vi "Limit range based on sensors.vi"(4 "Position":dbl, 6 "Position Max":dbl, 7 "min speed":dbl=-0.1 format="%#_13g", 8 "BottomDist":dbl=inf, 9 "Bottom SW":bool, 10 "Top SW":bool, 11 "output range in":cluster{"output high":dbl, "output low":dbl}) -> (3 "output range out":cluster{"output high":dbl, "output low":dbl})   [LabVIEW 2019]
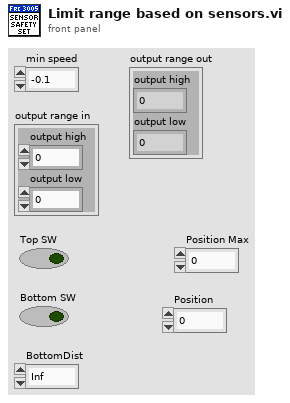
[diagram p1: front panel]
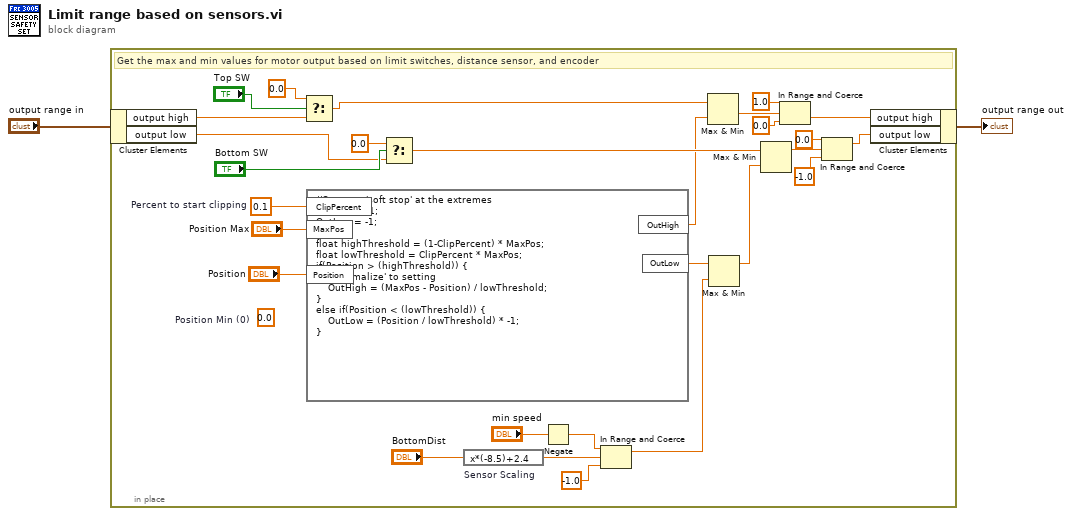
[diagram p0: block diagram]
diagram:
  n1 = in-place {
    w19 = 0.1  # Percent to start clipping
    (unwired) 0.0  # Position Min (0)
    # "Get the max and min values for motor output based on limit switches, distance sensor, and encoder"
    n2 = in-place-cluster #1("output range in") -> ("output high"=w26:dbl, "output low"=w25:dbl)
    n3 = Select(t=0.0, s="Top SW", f=w26) -> (s? t:f=w12:dbl)
    n4 = formula code="//Create a 'soft stop' at the extremes\nOutHigh = 1;\nOutLow = -1;\n\nfloat highThreshold = (1-ClipPercent) * MaxPos;\nfloat lowThreshold = ClipPercent * MaxPos;\nif(Position > (highThreshold)) {\n    //'normalize' to setting\n    OutHigh = (MaxPos - Position) / lowThreshold;\n}\nelse if(Position < (lowThreshold)) {\n    OutLow = (Position / lowThreshold) * -1;\n}"("MaxPos"="Position Max", "ClipPercent"=w19, "Position"="Position") -> ("OutHigh"=w13:dbl, "OutLow"=w16:dbl)
    n5 = Select(t=0.0, s="Bottom SW", f=w25) -> (s? t:f=w14:dbl)
    n6 = expression code="x*(-8.5)+2.4" "Sensor Scaling"("BottomDist") -> (w20:dbl)
    n7 = Negate(x="min speed") -> (-x=w22:dbl)
    n8 = In Range and Coerce(upper limit=w22, x=w20, lower limit=-1.0) -> (coerced(x)=w15:dbl)  [unwired: 1 out]
    n9 = Max & Min(x=w12, y=w13) -> (min(x,y)=w11:dbl)  [unwired: 1 out]
    n10 = Max & Min(x=w16, y=w15) -> (max(x,y)=w9:dbl)  [unwired: 1 out]
    n11 = Max & Min(x=w14, y=w9) -> (max(x,y)=w10:dbl)  [unwired: 1 out]
    n12 = In Range and Coerce(upper limit=1.0, x=w11, lower limit=0.0) -> (coerced(x)=w8:dbl)  [unwired: 1 out]
    n13 = In Range and Coerce(upper limit=0.0, x=w10, lower limit=-1.0) -> (coerced(x)=w5:dbl)  [unwired: 1 out]
    n14 = in-place-cluster #1("output high"=w8, "output low"=w5) -> (→"output range out":cluster{"output high":dbl, "output low":dbl})
  }
